vi "MARKET (SubVI).vi"() -> (2 "CRUDE OIL":dbl, 3 "USD TO RM":dbl)   [LabVIEW 2020]
panel:
  out "before substring":string
  out "match substring":string
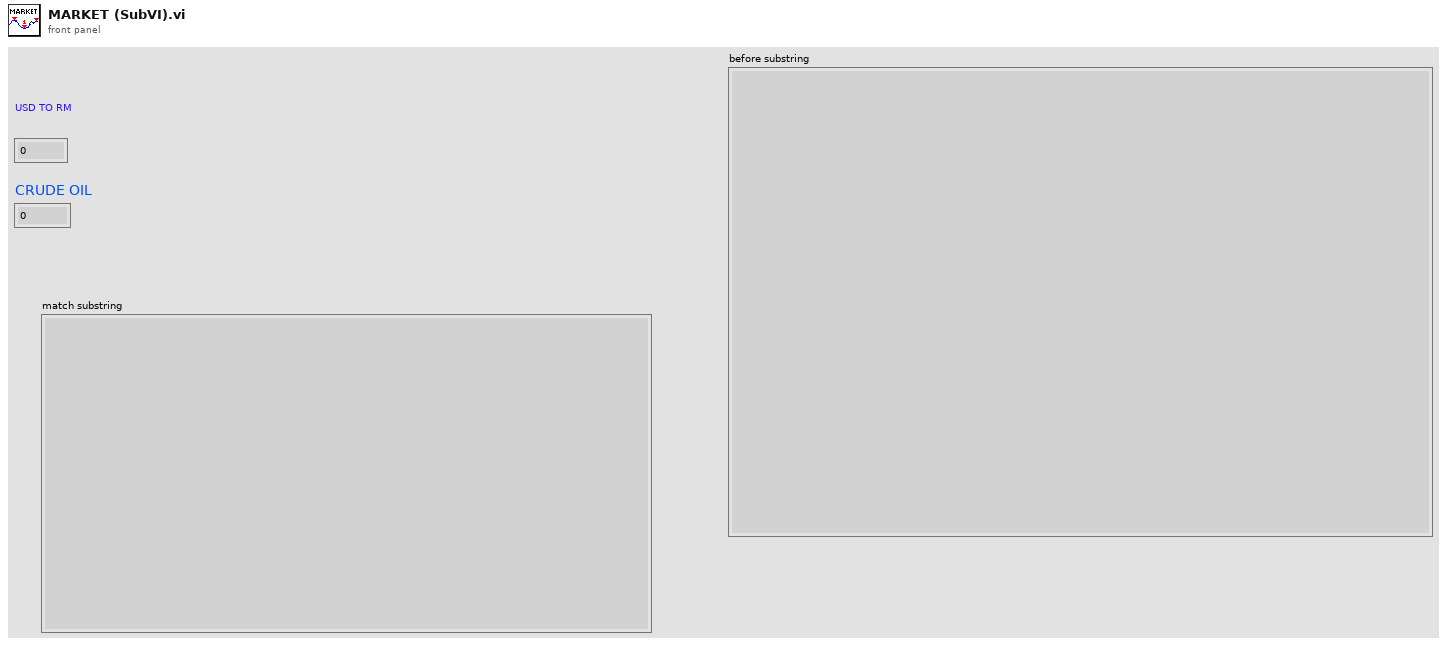
[diagram p1: front panel]
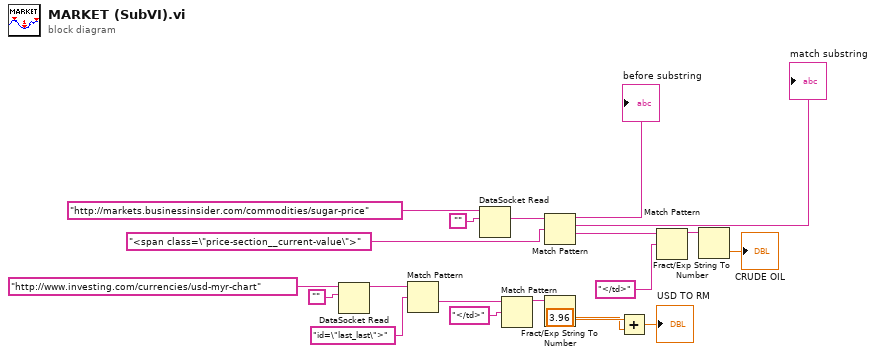
[diagram p0: block diagram]
diagram:
  n1 = DataSocket Read(10:"", 11:"http://www.investing.com/currencies/usd-myr-chart" ("connection in")) -> (3:w13:string)  [unwired: 3 in, 6 out]
  n2 = Match Pattern(string=w13, regular expression="id=\"last_last\">") -> (after substring=w15:string)  [unwired: 1 in, 3 out]
  n3 = DataSocket Read(10:"", 11:"http://markets.businessinsider.com/commodities/sugar-price") -> (2:w5:string)  [unwired: 3 in, 6 out]
  n4 = Match Pattern(string=w15, regular expression="</td>") -> (before substring=w17:string)  [unwired: 1 in, 3 out]
  n5 = Match Pattern(string=w5, regular expression="<span class=\"price-section__current-value\">") -> (before substring=→"before substring":string, match substring=→"match substring":string, after substring=w7:string)  [unwired: 1 in, 1 out]
  n6 = Fract/Exp String To Number(string=w17) -> (number=w19:dbl)  [unwired: 3 in, 1 out]
  n7 = Add(x=w19, y=3.96) -> (x+y=→"USD TO RM":dbl)
  n8 = Match Pattern(string=w7, regular expression="</td>") -> (before substring=w9:string)  [unwired: 1 in, 3 out]
  n9 = Fract/Exp String To Number(string=w9) -> (number=→"CRUDE OIL":dbl)  [unwired: 3 in, 1 out]
